vi "Receive.vi"(7 "Actor":refnum<class "Actor.lvclass">) -> (0 "Error out":errorcluster, 2 "Msg":refnum<class "Msg.lvclass">)   [LabVIEW 2025, in "jettl.lvlib" / "Transport.lvlib"]
uses:
  Transport.lvlib
  Actor/Actor/Actor.lvclass
  Msg/Msg.lvclass
  Queue Transport/Queue Transport.lvclass
  Attributes/Attributes/Attributes.lvclass
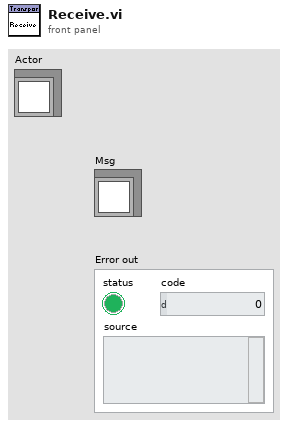
[diagram p1: front panel]
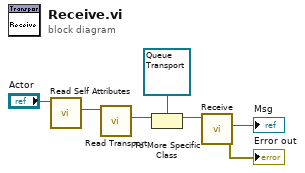
[diagram p0: block diagram]
diagram:
  n1 = call-dynamic "Read Self Attributes.vi"("Actor in"="Actor") -> ("Self Attributes"=w7:refnum<class "Attributes.lvclass">)  [unwired: 10 in]
  n2 = call-dynamic "Read Transport.vi"("Attributes in"=w7) -> ("Transport"=w5:refnum<class "Transport.lvclass">)  [unwired: 10 in]
  n3 = To More Specific Class(target class=refnum<class "Queue Transport.lvclass"> refnum ("jettl.lvlib:Transport.lvlib:Queue Transport.lvclass"), reference=w5) -> (specific class reference=w3:refnum<class "Queue Transport.lvclass">)  [unwired: 1 in, 1 out]
  n4 = call "Receive.vi"("Queue Transport in"=w3) -> ("Error out"=→"Error out":errorcluster, "Msg"=→"Msg":refnum<class "Msg.lvclass">)  [unwired: 9 in]
